vi "coulbourn-sound.vi"() -> ()   [LabVIEW 2012]
panel:
  in  "Trials completed":i32(slide) scale=0.0..60.0
  out "Waiting for trigger":bool
  out "Stimulus List File Path 3":path
  in  "OK Button 3":bool
  out "Stimulus List File Path 2":path
  in  "OK Button 2":bool
  in  "OK Button":bool
  in  "Trial Randomization":enum32{"50% exactly", "Radio Selection 2"}(radio)
  in  "Stims 2":dbl[][](array[numeric])
  in  "Stims 2 -- Colbourn Target String":string
  in  "Generate 3":bool
  in  "Stims 1 -- Colbourn Target String":string
  in  "Total Trials":dbl
  in  "Stims 1":dbl[][](array[numeric])
  in  "Stimulus List":dbl[][](array[numeric])
  in  "Generate 2":bool
  in  "Generate":bool
  # "Stim Type, Duration, Param 1, Param 2, Param 3, Param 4"
  # "Stim Type, Duration, Param 1, Param 2, Param 3, Param 4"
  # "Target, Stim Type, Duration, Param 1, Param 2, Param 3, Param 4"
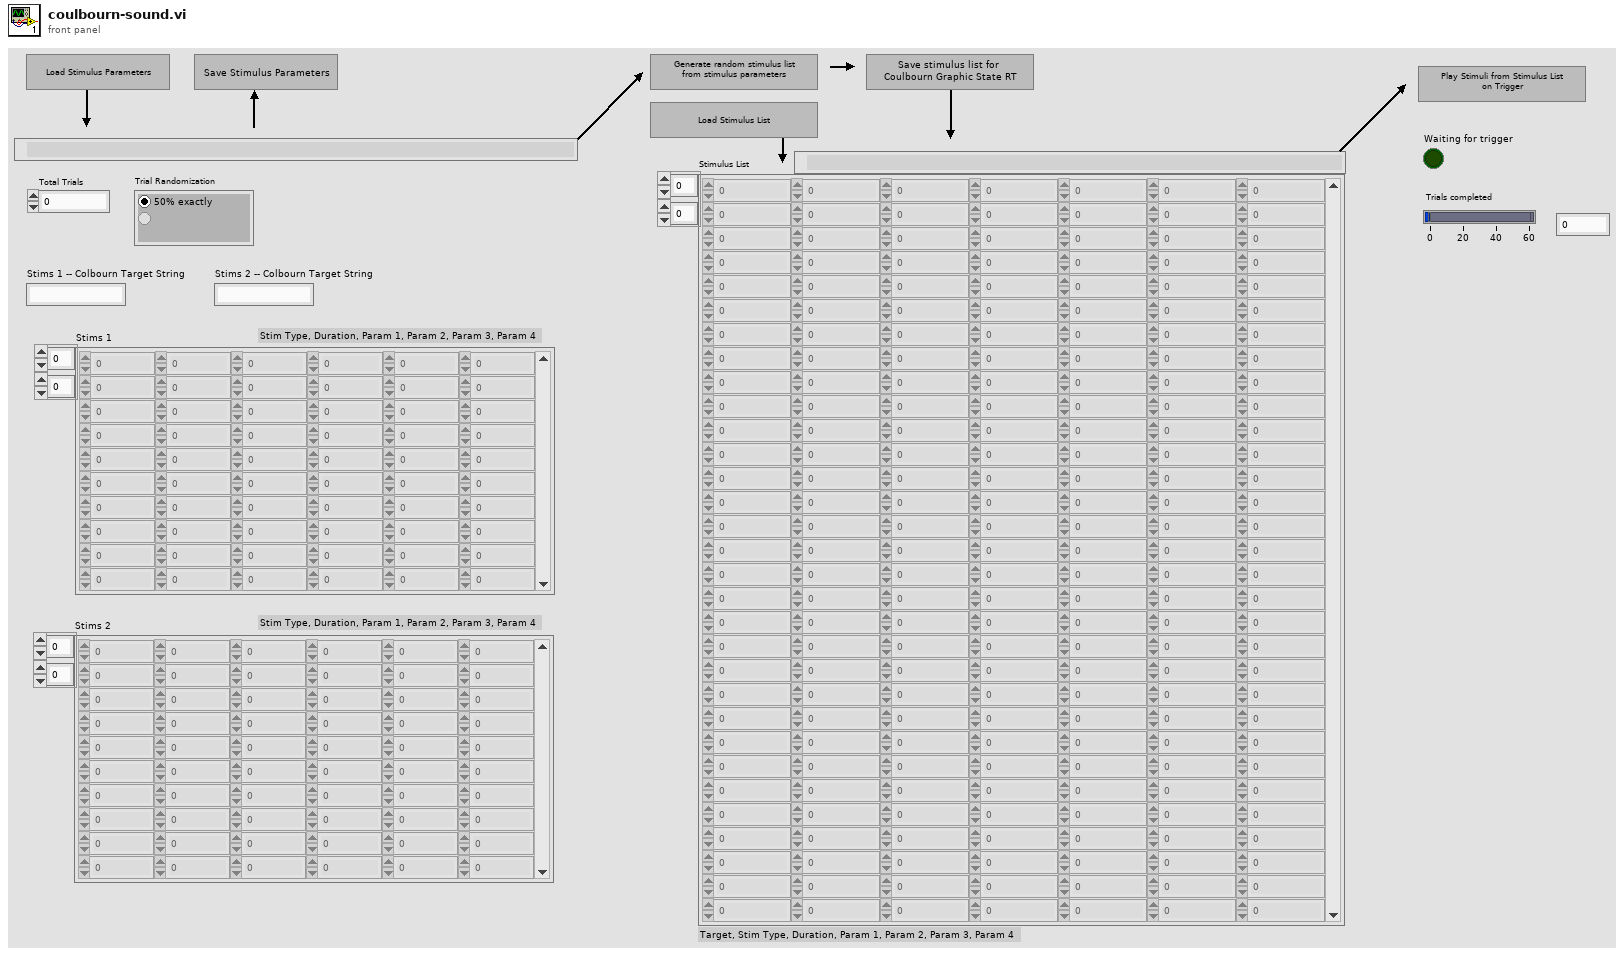
[diagram p1: front panel]
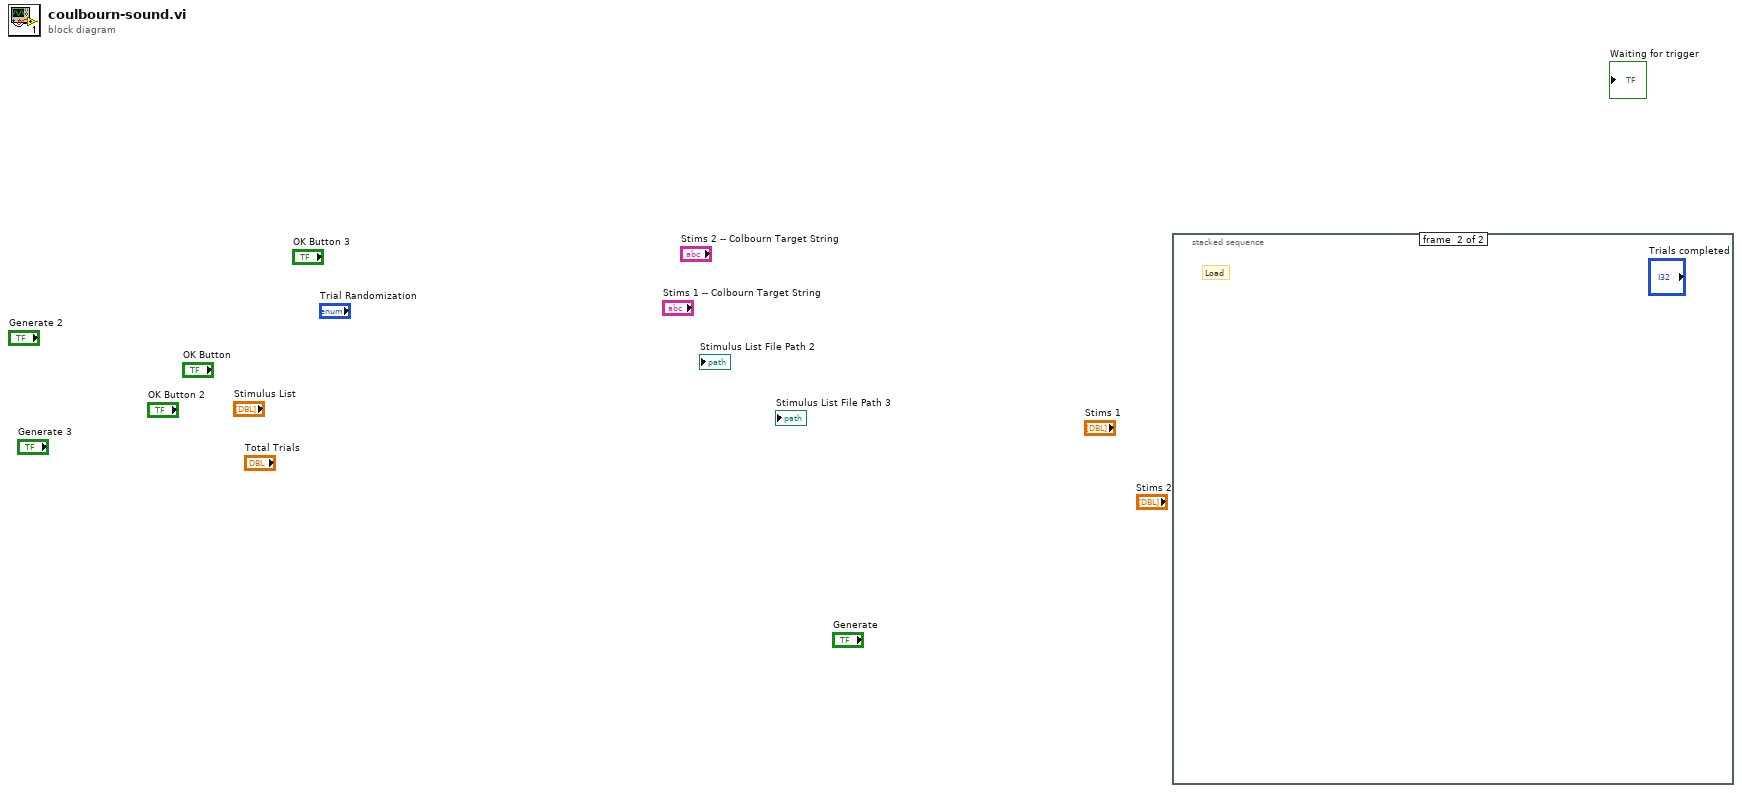
[diagram p0: block diagram]
diagram:
  n1 = stacked-sequence {
    frame #0 {
      # "Initialization"
    }
    frame #1 {
      # "Load"
    }
  }
